vi "Add Zenoh Error Core.vi"(8 "error in (no error)":errorcluster, 10 "String to Append":string, 11 "Error":T1) -> (0 "error out":errorcluster)   [LabVIEW 2021, in "Zenoh.lvclass"]
uses:
  Zenoh.lvclass
  Zenoh.lvclass/Zenoh.ctl
  <vilib>/CIF Foundation/CIF Utilities/Errors/Errors_CIF_U.lvlib
  typedef/Zenoh Errors.ctl
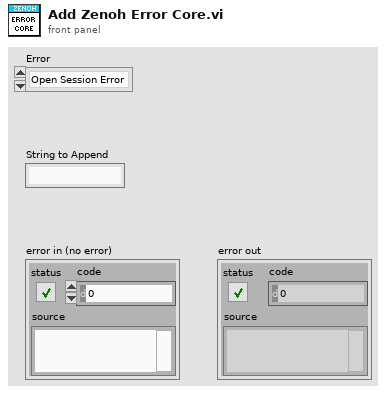
[diagram p1: front panel]
types:
  T1 = typedef "Zenoh.lvclass/Zenoh Errors.ctl" = enum16{"Open Session Error", "Open Subscription Error", "Declare Liveliness", "Query Keys", "File Error", "JSON Error", "Zenoh Runtime"}
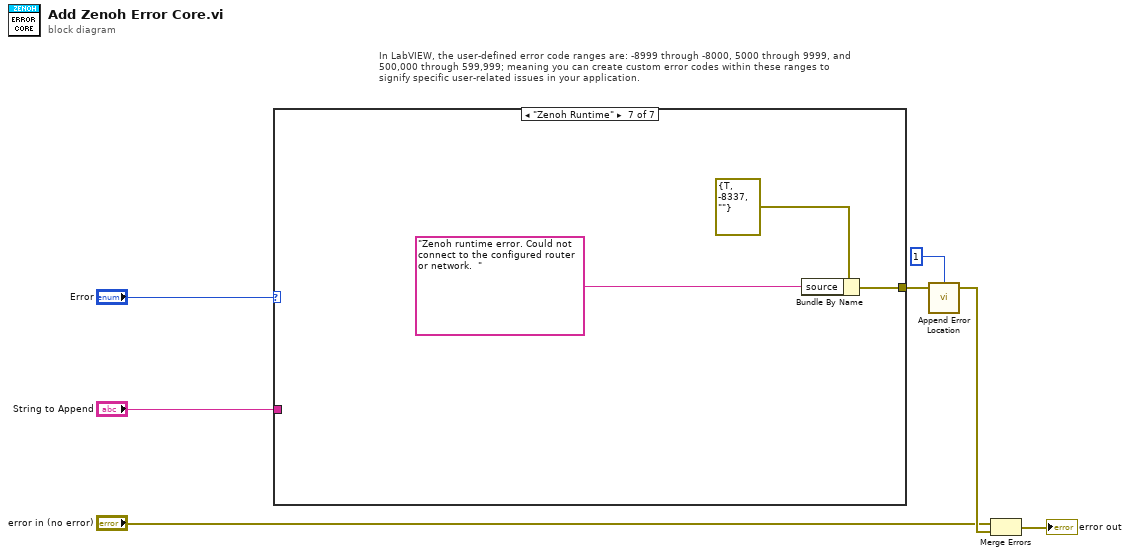
[diagram p0: block diagram]
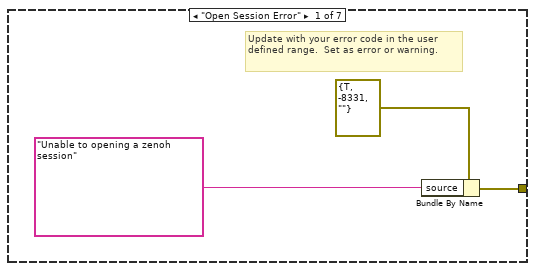
[diagram p2: hidden frame]
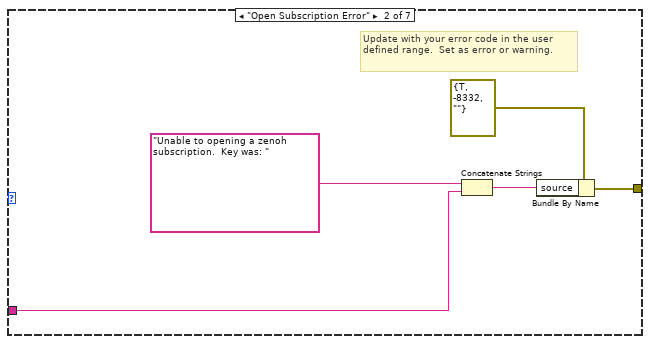
[diagram p3: hidden frame]
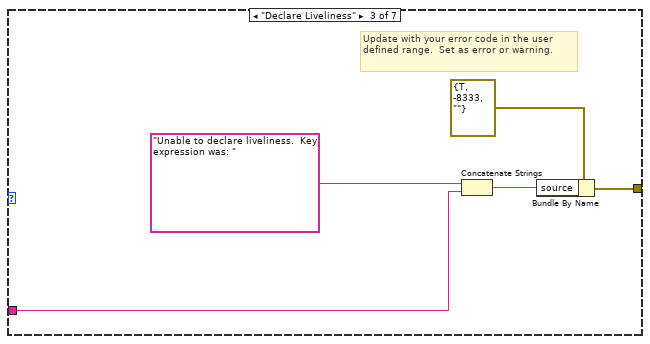
[diagram p4: hidden frame]
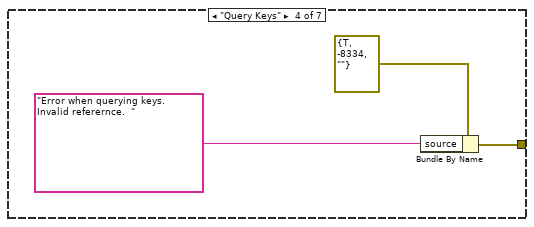
[diagram p5: hidden frame]
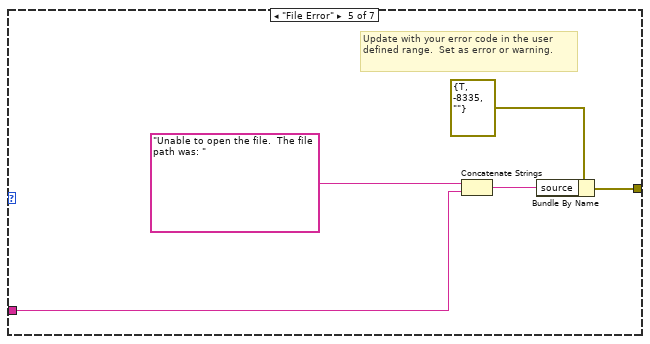
[diagram p6: hidden frame]
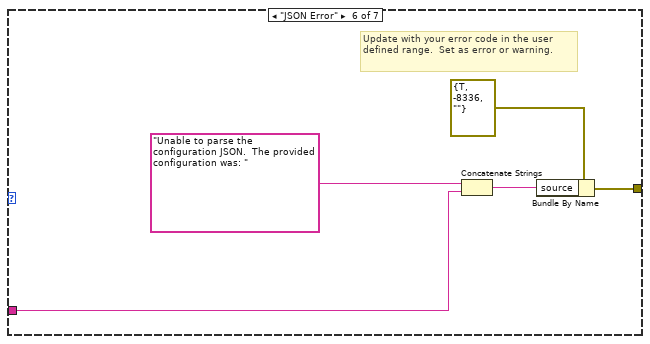
[diagram p7: hidden frame]
diagram:
  # "In LabVIEW, the user-defined error code ranges are: -8999 through -8000, 5000 through 9999, and 500,000 through 599,999; meaning you can create custom error codes within these ranges to signify specific user-related issues in your application."
  n1 = case shown="\"Zenoh Runtime\"" "Error" {
    tunnel: "String to Append" -> [_ w11 w16 _ w24 w29 _]
    tunnel: [w9 w14 w19 w22 w27 w32 w35] -> w6
    frame "Open Session Error" {
      # "Update with your error code in the user defined range.  Set as error or warning."
      n2 = Bundle By Name(cluster=errorcluster {"status"=TRUE, "code"=-8331, "source"=""} ("Invalid ID"), "source"="Unable to opening a zenoh session") -> (w9:errorcluster)
    }
    frame "Open Subscription Error" {
      # "Update with your error code in the user defined range.  Set as error or warning."
      n3 = Concatenate Strings("Unable to opening a zenoh subscription.  Key was: " ("source"), w11) -> (w12:string)
      n4 = Bundle By Name(cluster=errorcluster {"status"=TRUE, "code"=-8332, "source"=""} ("Invalid ID"), "source"=w12) -> (w14:errorcluster)
    }
    frame "Declare Liveliness" {
      # "Update with your error code in the user defined range.  Set as error or warning."
      n5 = Concatenate Strings("Unable to declare liveliness.  Key expression was: " ("source"), w16) -> (w17:string)
      n6 = Bundle By Name(cluster=errorcluster {"status"=TRUE, "code"=-8333, "source"=""} ("Invalid ID"), "source"=w17) -> (w19:errorcluster)
    }
    frame "Query Keys" {
      n7 = Bundle By Name(cluster=errorcluster {"status"=TRUE, "code"=-8334, "source"=""} ("Invalid ID"), "source"="Error when querying keys.  Invalid referernce.  ") -> (w22:errorcluster)
    }
    frame "File Error" {
      # "Update with your error code in the user defined range.  Set as error or warning."
      n8 = Concatenate Strings("Unable to open the file.  The file path was: " ("source"), w24) -> (w25:string)
      n9 = Bundle By Name(cluster=errorcluster {"status"=TRUE, "code"=-8335, "source"=""} ("Invalid ID"), "source"=w25) -> (w27:errorcluster)
    }
    frame "JSON Error" {
      # "Update with your error code in the user defined range.  Set as error or warning."
      n10 = Concatenate Strings("Unable to parse the configuration JSON.  The provided configuration was: " ("source"), w29) -> (w30:string)
      n11 = Bundle By Name(cluster=errorcluster {"status"=TRUE, "code"=-8336, "source"=""} ("Invalid ID"), "source"=w30) -> (w32:errorcluster)
    }
    frame "Zenoh Runtime" {
      n12 = Bundle By Name(cluster=errorcluster {"status"=TRUE, "code"=-8337, "source"=""} ("Invalid ID"), "source"="Zenoh runtime error. Could not connect to the configured router or network.  ") -> (w35:errorcluster)
    }
  }
  n13 = call <vilib>:"Append Error Location.vi"("error in (no error)"=w6, "Chain Depth"=1) -> ("error out"=w7:errorcluster)  [unwired: 3 in]
  n14 = Merge Errors("error in (no error)", w7) -> (→"error out":errorcluster)
